vi "GetAncestorChain.vi"(8 "error in (no error)":errorcluster, 11 "reference in":refnum<class "SwitchBase.lvclass">) -> (0 "error out":errorcluster, 1 "Chain Out":string[](array[string]), 2 "PPL? Out":bool[](array[boolean]), 3 "reference out":refnum<class "SwitchBase.lvclass">)   [LabVIEW 2022 SP3, in "SwitchBase.lvlib" / "SwitchBase.lvclass"]
uses:
  SwitchBase.lvclass
  Components/ViPER.lvlibp/ViPER.lvclass
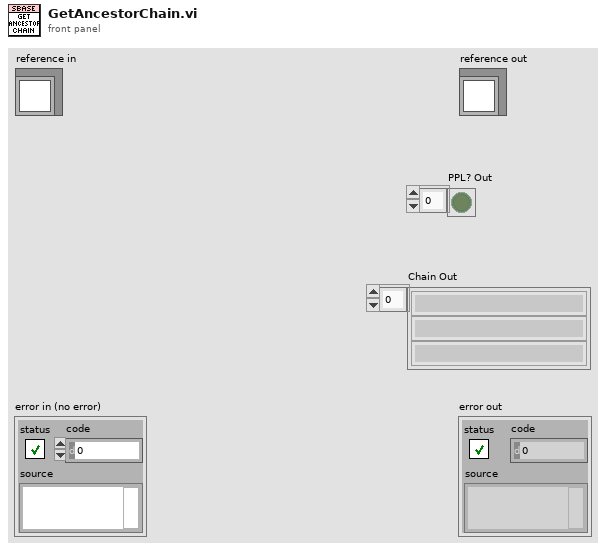
[diagram p1: front panel]
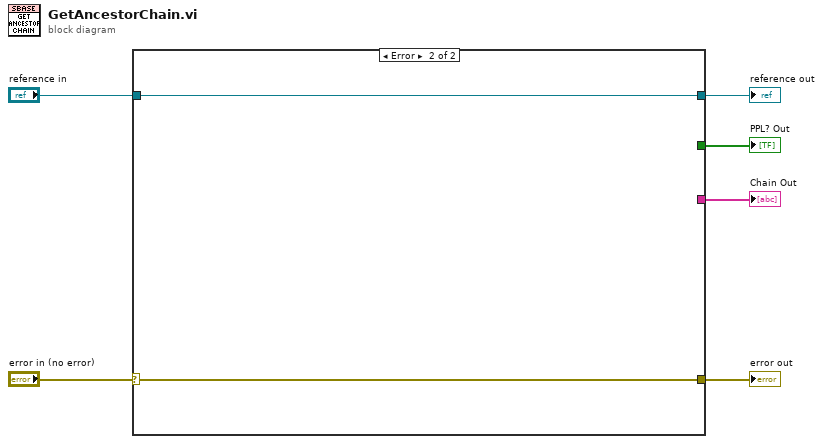
[diagram p0: block diagram]
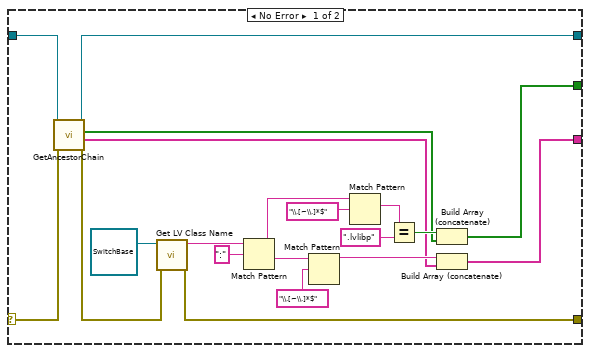
[diagram p2: hidden frame]
diagram:
  n1 = case shown="Error" "error in (no error)" {
    selector: "error in (no error)" -> [w13 w28]
    tunnel: [w7 w28] -> w5
    tunnel: "reference in" -> [w14 w27]
    tunnel: [w25 w27] -> w3
    tunnel: [w8 _] -> w2
    tunnel: [w9 _] -> w1
    frame No Error {
      n2 = call-parent "GetAncestorChain.vi"("error in (no error)"=w13, "reference in"=w14) -> ("error out"=w12:errorcluster, "Chain Out"=w11:string[], "PPL? Out"=w10:bool[], "reference out"=w25:refnum<class "SwitchBase.lvclass">)  [unwired: 6 in]
      n3 = call <vilib>:"Get LV Class Name.vi"("error in (no error)"=w12, "object"=refnum<class "SwitchBase.lvclass"> refnum ("reference in")) -> ("error out"=w7:errorcluster, "class name"=w17:string)  [unwired: 8 in]
      n4 = Match Pattern(string=w17, regular expression=":") -> (before substring=w22:string, after substring=w20:string)  [unwired: 1 in, 2 out]
      n5 = Match Pattern(string=w20, regular expression="\\.[~\\.]*$") -> (before substring=w16:string)  [unwired: 4 out]
      n6 = Match Pattern(string=w22, regular expression="\\.[~\\.]*$") -> (match substring=w23:string)  [unwired: 4 out]
      n7 = Equal?(x=w23, y=".lvlibp") -> (x = y?=w15:bool)
      n8 = Build Array (concatenate)(w15, w10) -> (w9:bool[])
      n9 = Build Array (concatenate)(w16, w11) -> (w8:string[])
    }
    frame Error {
    }
  }
  "error out" <- w5
  "reference out" <- w3
  "Chain Out" <- w2
  "PPL? Out" <- w1
